vi "Exp Avg Sound Level (decimated).vi"(0 "scaled signal [EU]":dbl[](array[numeric]) format="%.2f", 1 "sampling frequency [Hz]":dbl=10000.0 format="%.2f", 2 "decimating factor":i32=1 min=1 step=1, 3 "weighting filter":T1(ring), 4 "type":enum16{"Type 0", "Type 1"}(ring)=enum."Type 1", 5 "channel info":T2={"sensor sensitivity [mV/EU]"=1000.0, "engineering units"=1, "dB reference [EU]"=1.0, "custom label"="EU", "weighting filter"=0, "pregain [dB]"=0.0} {"pregain [dB]" format="%.2f"; "weighting filter" items=["Linear", "A-weighting", "B-weighting", "C-weighting", "ITU-R 468-4", "Dolby", "CCITT", "C-message"]; "dB reference [EU]" format="%^.1e"; "engineering units" items=["custom..."=0, "V"=1, "A"=21, "Pa"=2, "N"=20, "g"=3, "m/s^2"=4, "m/s"=5, "m"=6, "mm/s"=12, "mm"=13, "microns/s"=14, "microns"=15, "in/s^2"=7, "in/s"=8, "in"=9, "mils/s"=10, "mils"=11, "rad/s^2"=16, "rad/s"=17, "rad"=18, "strain"=19]; "sensor sensitivity [mV/EU]" format="%.2f"}, 6 "exponential mode":enum16{"Slow", "Fast", "Impulse", "Custom"}(ring)=enum."Fast", 7 "weighting filter init/cont (init:F)":bool, 8 "time constant [ms]":dbl=125.0 format="%.2f", 9 "exp avg init/cont (init:F)":bool) -> (13 "weighting conflict":bool, 14 "exp avg sound level [dB EU] (decimated)":dbl[](array[numeric]) format="%.2f", 15 "unit label":string, 16 "max freq within tolerances [Hz]":dbl format="%.2f", 17 "new time period [ms]":dbl=0.0001 format="%.2f", 18 "actual time constant [ms]":dbl=125.0 format="%.2f", 19 "improper decimating factor":bool)   [LabVIEW 2017]
doc: "Computes the exponential averaged sound level of the input signal X, based on the selected exponential averaging mode, and decimates this sound level by the selected decimating factor. Choose a decimating factor to generate a new sampling frequency in accordance with the Shannon Sampling Theorem to avoid aliasing problems. This means that the new time period must not exceed half the actual time constant."
uses:
  <vilib>/addons/Sound and Vibration/compatibility/Controls/svl_Channel Info.ctl
  <vilib>/addons/Sound and Vibration/compatibility/Controls/svl_Engineering Units Text Ring.ctl
  <vilib>/addons/Sound and Vibration/compatibility/Controls/svl_Weighting Filter Text Ring.ctl
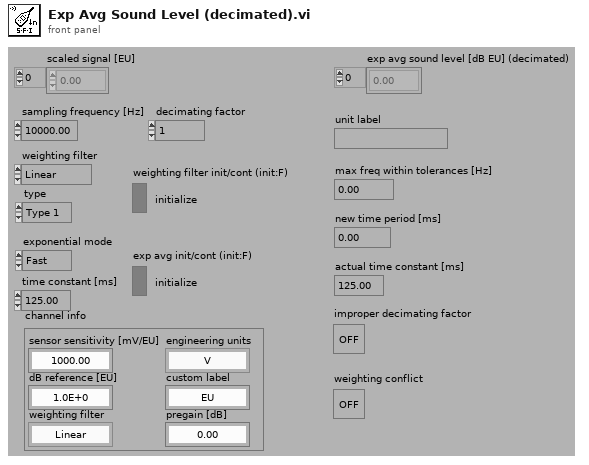
[diagram p1: front panel]
types:
  T1 = enum16{"Linear", "A-weighting", "B-weighting", "C-weighting"}
  T2 = typedef "svl_Channel Info.ctl" = cluster{"sensor sensitivity [mV/EU]":dbl, "engineering units":T3, "dB reference [EU]":dbl, "custom label":string, "weighting filter":T4, "pregain [dB]":dbl}
  T3 = typedef "svl_Engineering Units Text Ring.ctl" = u16
  T4 = typedef "svl_Weighting Filter Text Ring.ctl" = u16
  T5 = cluster{"exponential averaging":dbl, "peak detector":dbl}
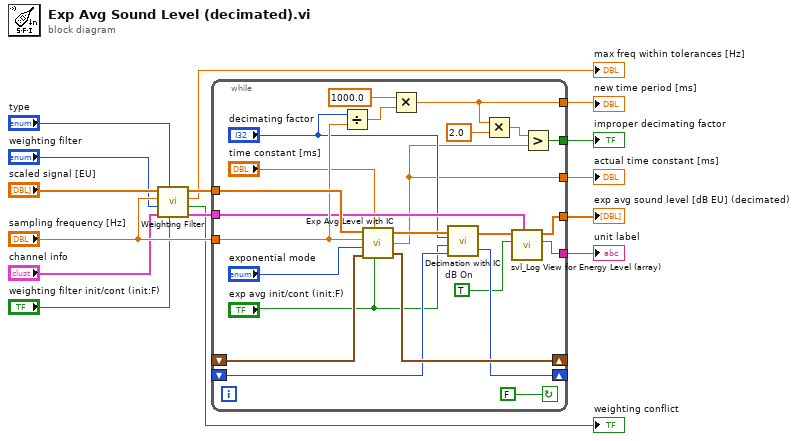
[diagram p0: block diagram]
diagram:
  n1 = call <vilib>:"Weighting Filter.vi"("weighting filter init/cont (init:F)"="weighting filter init/cont (init:F)", "type"="type", "channel info IN"="channel info", "weighting filter"="weighting filter", "sampling frequency [Hz]"="sampling frequency [Hz]", "scaled signal [EU]"="scaled signal [EU]") -> ("channel info OUT"=w5:T2, "weighting conflict"=→"weighting conflict":bool, "max freq within tolerances [Hz]"=→"max freq within tolerances [Hz]":dbl, "weighted signal [EU]"=w11:dbl[])
  n2 = while {
    tunnel: [w19] -> w1
    tunnel: w5 -> [w29]
    tunnel: [w30] -> w12
    tunnel: [w31] -> w13
    tunnel: [w17] -> w14
    tunnel: [w21] -> w15
    tunnel: w11 -> [w33]
    tunnel: "sampling frequency [Hz]" -> [w32]
    shift-left: _ -> [w35]
    shift-right: [w36] -> _
    shift-left: _ -> [w39]
    shift-right: [w38] -> _
    stop <- FALSE continue-if-true
    w28 = TRUE  # dB On
    n3 = Divide(x="decimating factor", y=w32) -> (x/y=w23:dbl)
    n4 = call <vilib>:"Exp Avg Level with IC.vi"("scaled signal [EU]"=w33, "time constant [ms]"="time constant [ms]", "sampling frequency [Hz]"=w32, "exponential mode"="exponential mode", "init/cont (init:F)"="exp avg init/cont (init:F)", "initial filter state"=w39) -> ("exp avg level [EU^2 rms]"=w37:dbl[], "actual time constant [ms]"=w17:dbl, "final filter state"=w38:T5)
    n5 = Multiply(x=1000.0, y=w23) -> (x*y=w21:dbl)
    n6 = call <vilib>:"Decimation with IC.vi"("initial decimation state"=w35, "init/cont (init:F)"="exp avg init/cont (init:F)", "decimating factor (1)"="decimating factor", "X"=w37) -> ("final decimation state"=w36:i32, "decimated X"=w34:dbl[])
    n7 = Multiply(x=w21, y=2.0) -> (x*y=w18:dbl)
    n8 = call <vilib>:"svl_Log View for Energy Level (array).vi"("channel info"=w29, "dB On (T)"=w28, "scaled signal"=w34) -> ("unit label"=w31:string, "log view scaled signal"=w30:dbl[])  [unwired: 6 in, 1 out]
    n9 = Greater?(x=w18, y=w17) -> (0:w19:bool)
  }
  "unit label" <- w13
  "new time period [ms]" <- w15
  "actual time constant [ms]" <- w14
  "exp avg sound level [dB EU] (decimated)" <- w12
  "improper decimating factor" <- w1
